vi "Measurement A.vi"(0 "Inputs":T1, 5 "Directory Path":path, 7 "First name":string, 9 "Last name":string, 11 "error in (no error)":errorcluster) -> (4 "Result":dbl, 6 "file or folder exists?":bool, 8 "Full name":string, 15 "error out":errorcluster)   [LabVIEW 2021]
uses:
  controls/Measurement Inputs.ctl
  controls/Offset value.ctl
  Reusables/controls/Username.ctl
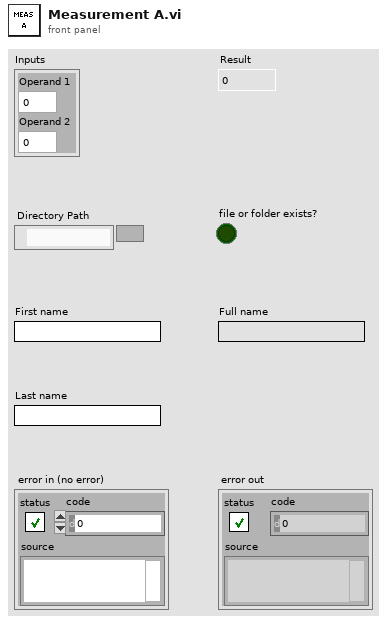
[diagram p1: front panel]
types:
  T1 = typedef "Measurement Inputs.ctl" = cluster{"Operand 1":dbl, "Operand 2":dbl}
  T2 = typedef "Username.ctl" = cluster{"First name":string, "Last name":string}
  T3 = typedef "Offset value.ctl" = cluster{"offset":dbl}
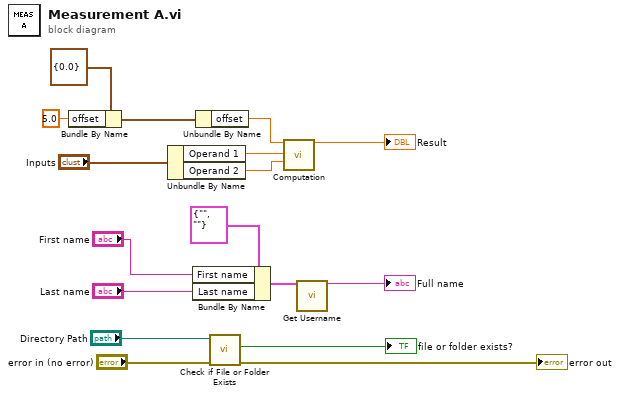
[diagram p0: block diagram]
diagram:
  n1 = Bundle By Name(cluster=T3 {"offset"=0.0}, "offset"=5.0) -> (w10:T3)
  n2 = Unbundle By Name("Inputs") -> ("Operand 1"=w16:dbl, "Operand 2"=w15:dbl)
  n3 = Bundle By Name(cluster=T2 {"First name"="", "Last name"=""} ("Name"), "First name"="First name", "Last name"="Last name") -> (w8:T2)
  n4 = Unbundle By Name(w10) -> ("offset"=w14:dbl)
  n5 = call <vilib>:"Check if File or Folder Exists.vi"("error in (no error)"="error in (no error)", "path"="Directory Path") -> ("error out"=→"error out":errorcluster, "file or folder exists?"=→"file or folder exists?":bool)  [unwired: 7 in, 1 out]
  n6 = call "Computation.vi"("offset"=w14, "Operand 1"=w16, "Operand 2"=w15) -> ("Result"=→"Result":dbl)  [unwired: 12 in]
  n7 = call "Get Username.vi"("Name"=w8) -> ("Full name"=→"Full name":string)  [unwired: 14 in]
